vi "NewGame.vi"(8 "error in (no error)":errorcluster, 10 "Engine in":refnum<class "Engine.lvclass">, 11 "MenuType (ChildObject)":refnum<class "Menu.lvclass">) -> (0 "error out":errorcluster, 2 "Engine out":refnum<class "Engine.lvclass">, 3 "Menu out":refnum<class "Menu.lvclass">)   [LabVIEW 2019, in "RT_Game.lvlib" / "Menu.lvclass"]
uses:
  Menu.lvclass
  C:/Users/FreshBob/Dropbox/VIs/myRIO_GameConsole/RT/RT_Game/Game/Game.lvclass
  Engine/Engine.lvclass
  Engine/Coordinate.ctl
  SnakeGame/SnakeGame.lvclass
  Pong/Pong.lvclass
  Bouncer/Bouncer.lvclass
  Color.ctl
  Engine/ScreenSide.ctl
  AboutScreen/AboutScreen.lvclass
  GPong/GPong.lvclass
  SnakeDemo/SnakeDemo.lvclass
  Game/Game.lvclass/Game.ctl
  Menu.lvclass/Menu.ctl
  Game/Write Singleplayer.vi
  Game/Game.lvclass
  RT_Game.lvlib
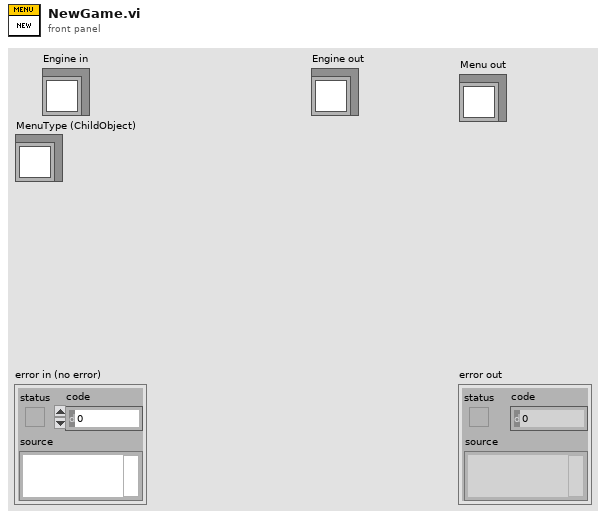
[diagram p1: front panel]
types:
  T1 = typedef "RT_Game.lvlib/Engine.lvclass/ScreenSide.ctl" = enum16{"up", "down", "left", "right", "none"}
  T2 = typedef "RT_Game.lvlib/Color.ctl" = fxp<+,3,3>
  T3 = typedef "RT_Game.lvlib/Engine.lvclass/Coordinate.ctl" = cluster{"x":dbl, "y":dbl}
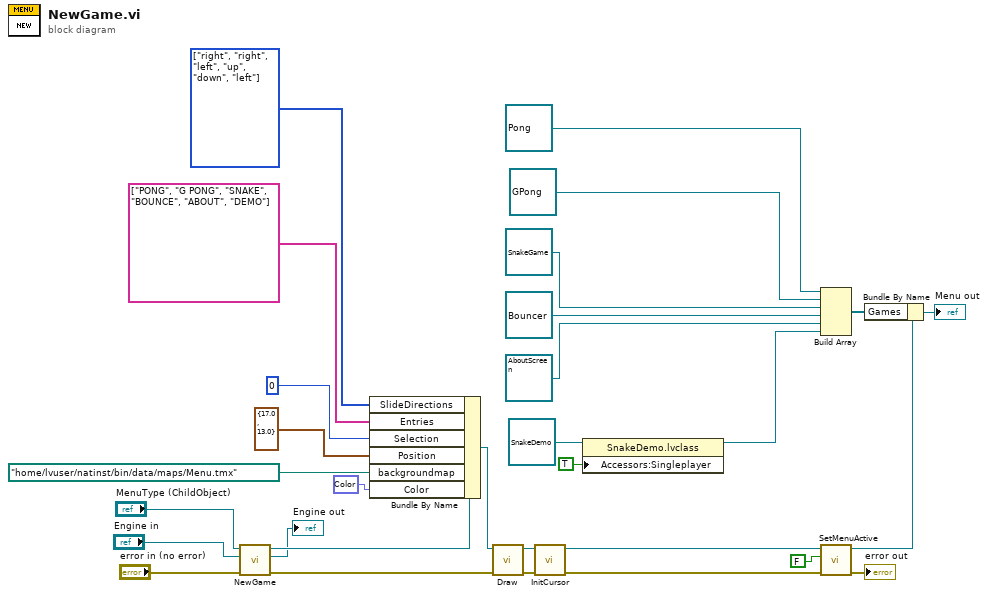
[diagram p0: block diagram]
diagram:
  w26 = T1[] [enum."right", enum."right", enum."left", enum."up", enum."down", enum."left"] items=["up", "down", "left", "right", "none"] ("SlideDirections")
  n1 = call-parent "NewGame.vi"("error in (no error)"="error in (no error)", "Engine in"="Engine in", "GameType (ChildObject)"="MenuType (ChildObject)") -> ("error out"=w9:errorcluster, "Engine out"=→"Engine out":refnum<class "Engine.lvclass">, "Game out"=w8:refnum<class "Menu.lvclass">)  [unwired: 6 in]
  n2 = Bundle By Name(cluster=w8, "SlideDirections"=w26, "Entries"=string[] ["PONG", "G PONG", "SNAKE", "BOUNCE", "ABOUT", "DEMO"], "Selection"=i8 0, "Position"=T3 {"x"=17.0, "y"=13.0}, "backgroundmap"=path "/home/lvuser/natinst/bin/data/maps/Menu.tmx" ("path to tmx-file (created with Tiles2D)"), "Color"=T2 1.0) -> (w16:refnum<class "Menu.lvclass">)
  n3 = call "Draw.vi"("error in (no error)"=w9, "Menu in"=w16) -> ("error out"=w15:errorcluster, "Menu out"=w18:refnum<class "Menu.lvclass">)  [unwired: 8 in]
  n4 = call "InitCursor.vi"("error in (no error)"=w15, "Menu in"=w18) -> ("error out"=w17:errorcluster, "Menu out"=w25:refnum<class "Menu.lvclass">)  [unwired: 8 in]
  n5 = property class="SnakeDemo.lvclass"(reference=refnum<class "SnakeDemo.lvclass"> refnum ("RT_Game.lvlib:SnakeDemo.lvclass"), "Accessors:Singleplayer"=TRUE ("Singleplayer")) -> (reference out=w2:refnum<class "SnakeDemo.lvclass">)  [unwired: 1 in, 1 out]
  n6 = Build Array(refnum<class "Pong.lvclass"> refnum ("RT_Game.lvlib:Pong.lvclass"), refnum<class "GPong.lvclass"> refnum ("RT_Game.lvlib:GPong.lvclass"), refnum<class "SnakeGame.lvclass"> refnum ("RT_Game.lvlib:Snake.lvclass"), refnum<class "Bouncer.lvclass"> refnum ("RT_Game.lvlib:Bouncer.lvclass"), refnum<class "AboutScreen.lvclass"> refnum ("RT_Game.lvlib:AboutScreen.lvclass"), w2) -> (w4:refnum<class "Game.lvclass">[])
  n7 = call "SetMenuActive.vi"("error in (no error)"=w17, "Active?"=FALSE, "Game in"=w25) -> ("error out"=→"error out":errorcluster, "Game out"=w28:refnum<class "Menu.lvclass">)  [unwired: 7 in]
  n8 = Bundle By Name(cluster=w28, "Games"=w4) -> (→"Menu out":refnum<class "Menu.lvclass">)
